vi "name search.vi"(9 "Value 2":string[][](array[string]), 10 "Value":string, 11 "Value 3":bool) -> (3 "User/Admin":string)   [LabVIEW 2019]
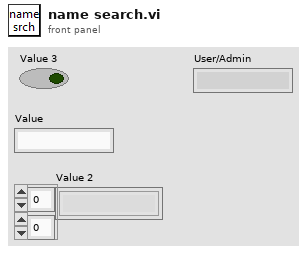
[diagram p1: front panel]
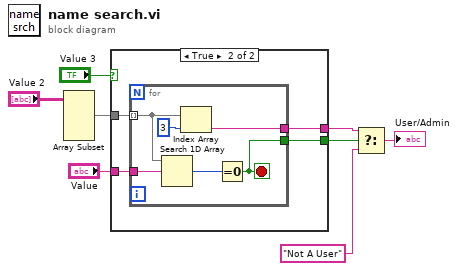
[diagram p0: block diagram]
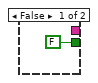
[diagram p2: hidden frame]
diagram:
  n1 = Array Subset(array="Value 2") -> (w7:string[][])  [unwired: 4 in]
  n2 = case shown="True" "Value 3" {
    tunnel: w7 -> [_ w13]
    tunnel: [_ w12] -> w3
    tunnel: [FALSE w11] -> w4
    tunnel: "Value" -> [_ w10]
    frame False {
    }
    frame True {
      n3 = for {
        tunnel: w13 -> [w19] mode=indexing
        tunnel: [w17] -> w12
        tunnel: [w15] -> w11
        tunnel: w10 -> [w14]
        stop <- w15 stop-if-true
        n4 = Search 1D Array(1D array=w19, element=w14) -> (index of element=w16:i32)  [unwired: 1 in]
        n5 = Index Array(array=w19, index=3) -> (element=w17:string)
        n6 = Equal To 0?(x=w16) -> (x = 0?=w15:bool)
      }
    }
  }
  n7 = Select(t=w3, s=w4, f="Not A User" ("User/Admin")) -> (s? t:f=→"User/Admin":string)
